vi "mean.vi"(11 "data in":T2) -> (3 "xyz":T1)   [LabVIEW 2019, in "Nano33BLE-TiltCompensationSupport.lvlib"]
uses:
  types/xyz_array.ctl
  types/xyz.ctl
  <vilib>/Analysis/baseanly.llb/Mean (DBL).vi
  Nano33BLE-TiltCompensationSupport.lvlib
  <vilib>/Analysis/NI_AALBase.lvlib
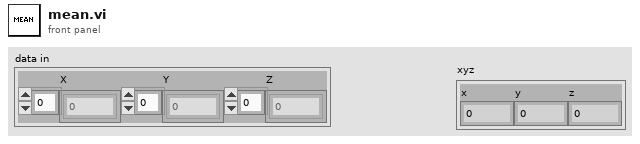
[diagram p1: front panel]
types:
  T1 = typedef "Nano33BLE-TiltCompensationSupport.lvlib/xyz.ctl" = cluster{"x":dbl, "y":dbl, "z":dbl}
  T2 = typedef "Nano33BLE-TiltCompensationSupport.lvlib/xyz_array.ctl" = cluster{"X":dbl[], "Y":dbl[], "Z":dbl[]}
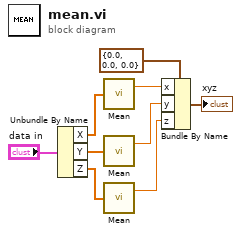
[diagram p0: block diagram]
diagram:
  n1 = Unbundle By Name("data in") -> ("X"=w8:dbl[], "Y"=w7:dbl[], "Z"=w6:dbl[])
  n2 = call-poly <vilib>:"Mean.vi"("X"=w8) -> ("mean"=w4:dbl)  [unwired: 1 out]
  n3 = call-poly <vilib>:"Mean.vi"("X"=w7) -> ("mean"=w3:dbl)  [unwired: 1 out]
  n4 = call-poly <vilib>:"Mean.vi"("X"=w6) -> ("mean"=w2:dbl)  [unwired: 1 out]
  n5 = Bundle By Name(cluster=T1 {"x"=0.0, "y"=0.0, "z"=0.0} ("xyz"), "x"=w4, "y"=w3, "z"=w2) -> (→"xyz":T1)
